vi "Climb Teleop Handler.vi"   [LabVIEW 2025]
types:
  T1 = typedef "WPI_JoystickDevRef.ctl" = cluster{"Device":T2}
  T2 = typedef "WPI_JoystickDeviceEnum.ctl" = enum16{"USB 0", "USB 1", "USB 2", "USB 3", "USB 4", "USB 5"}
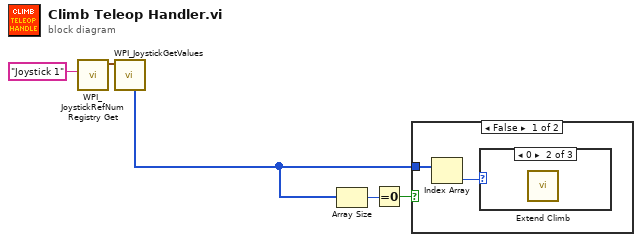
[diagram p0: block diagram]
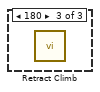
[diagram p3: hidden frame]
diagram:
  n1 = call <vilib>:"WPI_JoystickRefNum Registry Get.vi"("refnum name"="Joystick 1") -> ("JoystickDevRef"=w4:T1)  [unwired: 1 in, 9 out]
  n2 = call <vilib>:"WPI_JoystickGetValues.vi"("JoystickDevRef"=w4) -> ("POVs"=w1:i16[])  [unwired: 6 in, 4 out]
  n3 = Array Size(array=w1) -> (size(s)=w3:i32)
  n4 = Equal To 0?(x=w3) -> (x = 0?=w2:bool)
  n5 = case shown="False" w2 {
    tunnel: w1 -> [w6 _]
    frame False {
      n6 = Index Array(array=w6) -> (element=w7:i16)  [unwired: 1 in]
      n7 = case shown="0" w7 {
        frame -1, Default {
        }
        frame 0 {
          n8 = call "Extend Climb.vi"() -> ()  [unwired: 11 in, 1 out]
        }
        frame 180 {
          n9 = call "Retract Climb.vi"() -> ()  [unwired: 11 in, 1 out]
        }
      }
    }
    frame True {
    }
  }
